vi "Convert_String_to_TimeStamp.vi"(1 "date/time string":string) -> (0 "Resulting Time Stamp":timestamp)   [LabVIEW 2010]
doc: "This VI convert a date/time string back to a time stamp."
panel:
  # "This control should have data in the form:\n4/30/2004 7:48:47 PM"
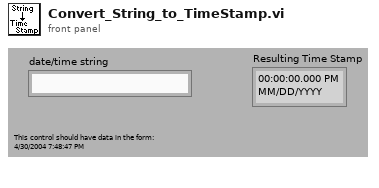
[diagram p1: front panel]
types:
  T1 = cluster{"second":i32, "minute":i32, "hour":i32, "day of month":i32, "month":i32, "year":i32, "day of week":i32, "day of year":i32, "is DST":i32}
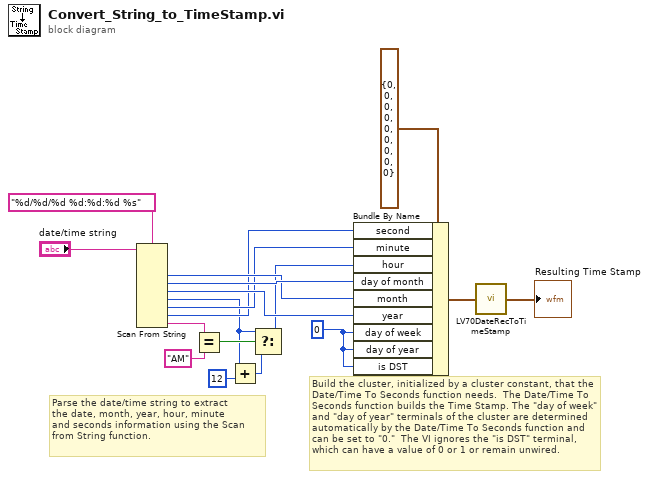
[diagram p0: block diagram]
diagram:
  w13 = 0
  # "Build the cluster, initialized by a cluster constant, that the Date/Time To Seconds function needs.  The Date/Time To Seconds function builds the Time Stamp. The \"day of week\" and \"day of year\" terminals of the cluster are determined automatically by the Date/Time To Seconds function and can be set to \"0.\"  The VI ignores the \"is DST\" terminal, which can have a value of 0 or 1 or remain unwired."
  # "Parse the date/time string to extract \nthe date, month, year, hour, minute \nand seconds information using the Scan\nfrom String function."
  n1 = Scan From String "Scan From String"(format string="%d/%d/%d %d:%d:%d %s", input string="date/time string") -> (output 1=w11:i32, output 2=w12:i32, output 3=w10:i32, output 4=w2:i32, output 5=w9:i32, output 6=w8:i32, output 7=w7:string)  [unwired: 9 in, 3 out]
  n2 = Equal?(x=w7, y="AM") -> (x = y?=w5:bool)
  n3 = Add(x=w2, y=12) -> (x+y=w3:i32)
  n4 = Select(t=w2, s=w5, f=w3) -> (s? t:f=w4:i32)
  n5 = Bundle By Name(cluster=T1 {"second"=0, "minute"=0, "hour"=0, "day of month"=0, "month"=0, "year"=0, "day of week"=0, "day of year"=0, "is DST"=0} ("date time rec"), "second"=w8, "minute"=w9, "hour"=w4, "day of month"=w12, "month"=w11, "year"=w10, "day of week"=w13, "day of year"=w13, "is DST"=w13) -> (w14:T1)
  n6 = call <vilib>:"LV70DateRecToTimeStamp.vi"("date time rec"=w14) -> ("Time Stamp"=→"Resulting Time Stamp":timestamp)
